vi "PathPlanner_PathFinder_IsWalkable.vi"(9 "S2":T1, 11 "S1":T1) -> (3 "IsWalkable":bool)   [LabVIEW 2019, in "PathPlanner24.lvlib"]
uses:
  TypeDef/PathPlannerFinderGridPosition.ctl
  PathPlanner_PathFinder_Globals.vi
  PathPlanner24.lvlib
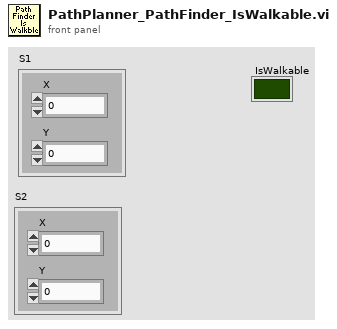
[diagram p1: front panel]
types:
  T1 = typedef "PathPlanner24.lvlib/PathPlannerFinderGridPosition.ctl" = cluster{"X":i32, "Y":i32}
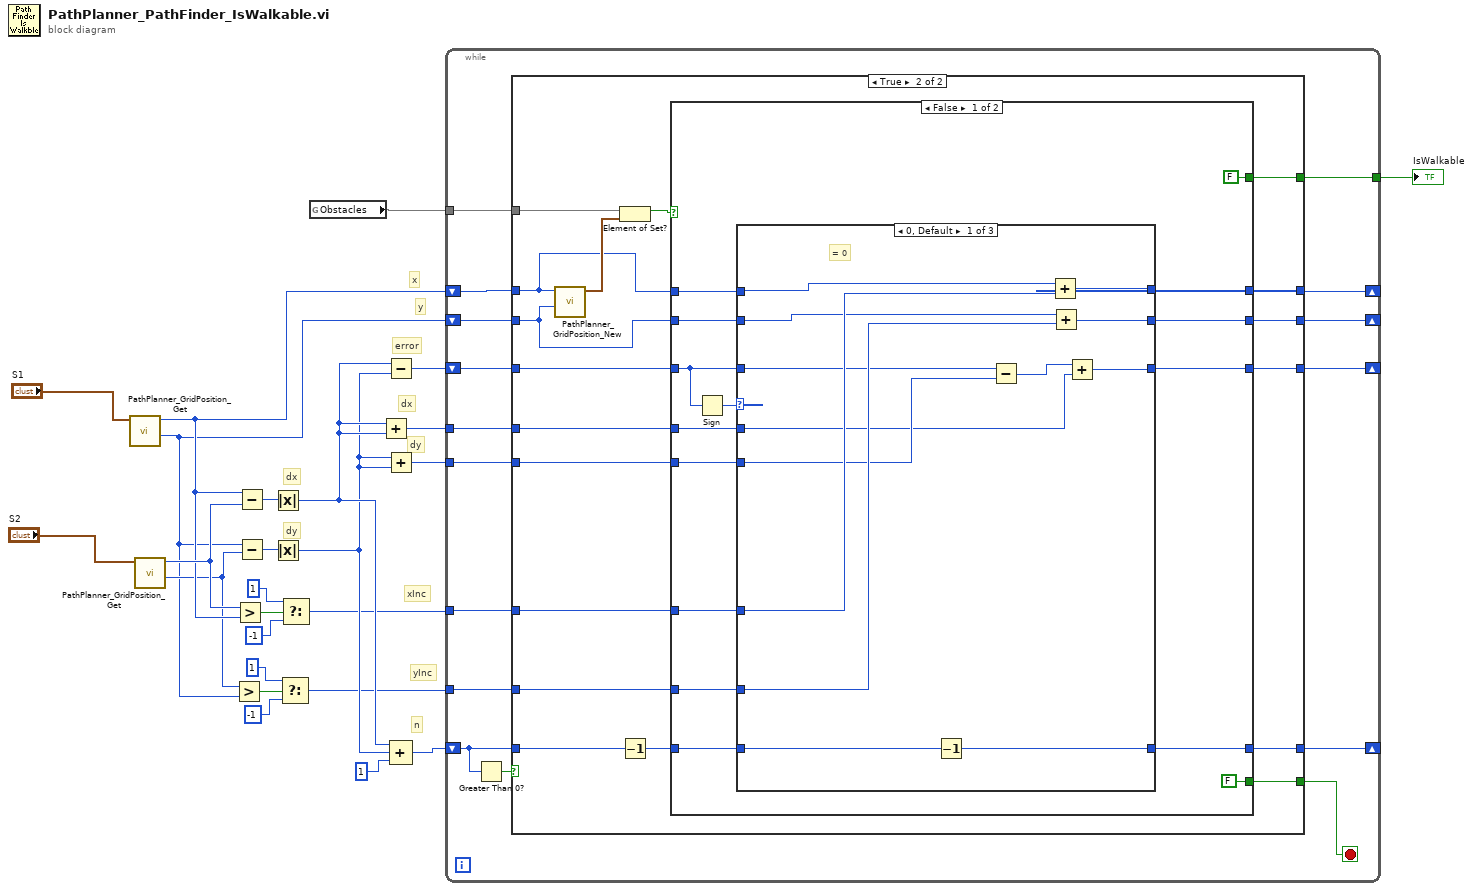
[diagram p0: block diagram]
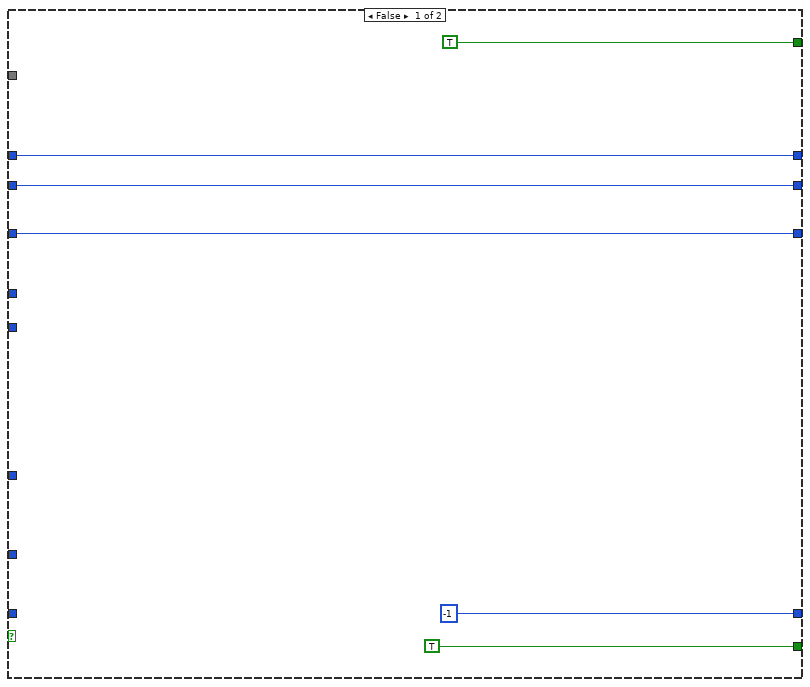
[diagram p2: hidden frame]
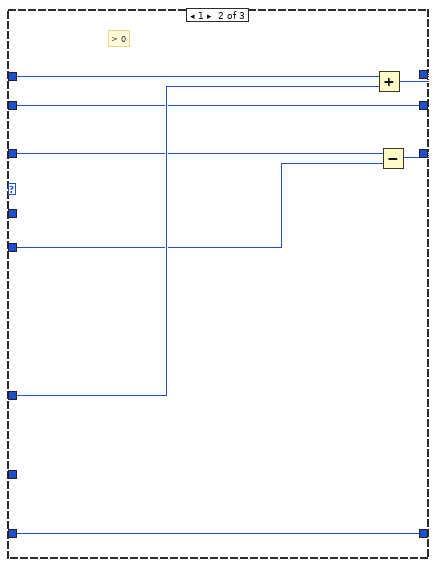
[diagram p3: hidden frame]
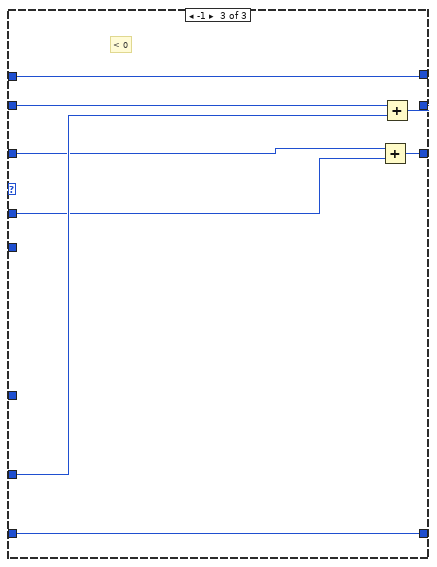
[diagram p4: hidden frame]
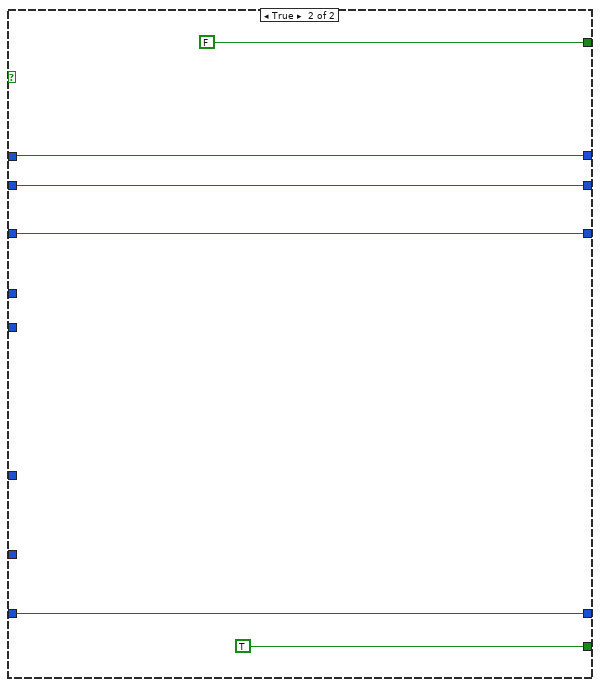
[diagram p5: hidden frame]
diagram:
  # "yInc"
  # "xInc"
  # "error"
  # "dy"
  # "dx"
  # "y"
  # "x"
  # "n"
  # "dy"
  # "dx"
  n1 = call "PathPlanner_GridPosition_Get.vi"("GridPosition"="S1") -> ("Y"=w3:i32, "X"=w10:i32)  [unwired: 9 in]
  n2 = call "PathPlanner_GridPosition_Get.vi"("GridPosition"="S2") -> ("Y"=w4:i32, "X"=w11:i32)  [unwired: 9 in]
  n3 = Greater?(x=w4, y=w3) -> (0:w7:bool)
  n4 = Greater?(x=w11, y=w10) -> (0:w12:bool)
  n5 = Subtract(x=w10, y=w11) -> (x-y=w23:i32)
  n6 = Subtract(x=w3, y=w4) -> (x-y=w22:i32)
  n7 = Absolute Value(x=w23) -> (abs(x)=w15:i32)
  n8 = Absolute Value(x=w22) -> (abs(x)=w14:i32)
  n9 = Select(t=1, s=w7, f=-1) -> (s? t:f=w1:i32)
  n10 = Select(t=1, s=w12, f=-1) -> (s? t:f=w2:i32)
  n11 = global read "PathPlanner_PathFinder_Globals.vi" "Obstacles"() -> (w17:set{T1})
  n12 = Add(x=w15, y=w15) -> (x+y=w18:i32)
  n13 = Subtract(x=w15, y=w14) -> (x-y=w13:i32)
  n14 = Add(x=w14, y=w14) -> (x+y=w19:i32)
  n15 = Compound Arithmetic op=ADD(w15, w14, 1 ("value")) -> (w21:i32)
  n16 = while {
    shift-right: [w34] -> _
    shift-left: w21 -> [w39]
    shift-right: [w33] -> _
    shift-left: w10 -> [w38]
    shift-right: [w32] -> _
    shift-left: w3 -> [w37]
    tunnel: w19 -> [w29]
    tunnel: w18 -> [w26]
    tunnel: w17 -> [w36]
    tunnel: [w35] -> w16
    shift-right: [w28] -> _
    shift-left: w13 -> [w31]
    tunnel: w2 -> [w30]
    tunnel: w1 -> [w27]
    stop <- w40 stop-if-true
    n17 = Greater Than 0?(x=w39) -> (x > 0?=w41:bool)
    n18 = case shown="True" w41 {
      tunnel: [TRUE w61] -> w40
      tunnel: w39 -> [_ w60]
      tunnel: w38 -> [w44 w56]
      tunnel: w37 -> [w43 w54]
      tunnel: w36 -> [_ w65]
      tunnel: [TRUE w62] -> w35
      tunnel: [-1 w58] -> w34
      tunnel: [w44 w57] -> w33
      tunnel: [w43 w55] -> w32
      tunnel: w31 -> [w42 w53]
      tunnel: w30 -> [_ w52]
      tunnel: w29 -> [_ w51]
      tunnel: [w42 w50] -> w28
      tunnel: w27 -> [_ w49]
      tunnel: w26 -> [_ w48]
      frame False {
      }
      frame True {
        n19 = call "PathPlanner_GridPosition_New.vi"("Y"=w54, "X"=w56) -> ("GridPosition"=w64:T1)  [unwired: 9 in]
        n20 = Element of Set?(10:w64, 11:w65) -> (3:w63:bool)
        n21 = Decrement(x=w60) -> (x-1=w59:i32)
        n22 = case shown="False" w63 {
          tunnel: [FALSE FALSE] -> w62
          tunnel: [FALSE TRUE] -> w61
          tunnel: w59 -> [w67 w113]
          tunnel: [w66 w113] -> w58
          tunnel: w56 -> [w79 w112]
          tunnel: [w77 w112] -> w57
          tunnel: w54 -> [w73 w111]
          tunnel: [w72 w111] -> w55
          tunnel: w53 -> [w76 w110]
          tunnel: w52 -> [w78 _]
          tunnel: w51 -> [w75 _]
          tunnel: [w74 w110] -> w50
          tunnel: w49 -> [w71 _]
          tunnel: w48 -> [w70 _]
          frame False {
            n23 = Sign(1:w76) -> (0:w80:i32)
            n24 = case shown="0, Default" w80 {
              tunnel: w79 -> [w93 w101 w103]
              tunnel: w78 -> [w92 w100 _]
              tunnel: [w91 w99 w103] -> w77
              tunnel: w76 -> [w87 w98 w106]
              tunnel: w75 -> [w86 w97 _]
              tunnel: [w83 w96 w104] -> w74
              tunnel: w73 -> [w90 w95 w109]
              tunnel: [w88 w95 w107] -> w72
              tunnel: w71 -> [w89 _ w108]
              tunnel: w70 -> [w84 _ w105]
              tunnel: w67 -> [w82 w94 w102]
              tunnel: [w81 w94 w102] -> w66
              frame 0, Default {
                # "= 0"
                n25 = Decrement(x=w82) -> (x-1=w81:i32)
                n26 = Subtract(x=w87, y=w86) -> (x-y=w85:i32)
                n27 = Add(x=w93, y=w92) -> (x+y=w91:i32)
                n28 = Add(x=w90, y=w89) -> (x+y=w88:i32)
                n29 = Add(x=w85, y=w84) -> (x+y=w83:i32)
              }
              frame 1 {
                # "> 0"
                n30 = Add(x=w101, y=w100) -> (x+y=w99:i32)
                n31 = Subtract(x=w98, y=w97) -> (x-y=w96:i32)
              }
              frame -1 {
                # "< 0"
                n32 = Add(x=w106, y=w105) -> (x+y=w104:i32)
                n33 = Add(x=w109, y=w108) -> (x+y=w107:i32)
              }
            }
          }
          frame True {
          }
        }
      }
    }
  }
  "IsWalkable" <- w16
